vi "Write Used DAQChannels.vi"(8 "error in (no error)":errorcluster, 10 "Used DAQChannels":tag[](array[tag]), 11 "SequencerConfig in":refnum<class "SequencerConfig.lvclass">) -> (0 "error out":errorcluster, 3 "SequencerConfig out":refnum<class "SequencerConfig.lvclass">)   [LabVIEW 2015, in "Sequencer.lvlib" / "SequencerConfig.lvclass"]
uses:
  SequencerConfig.lvclass
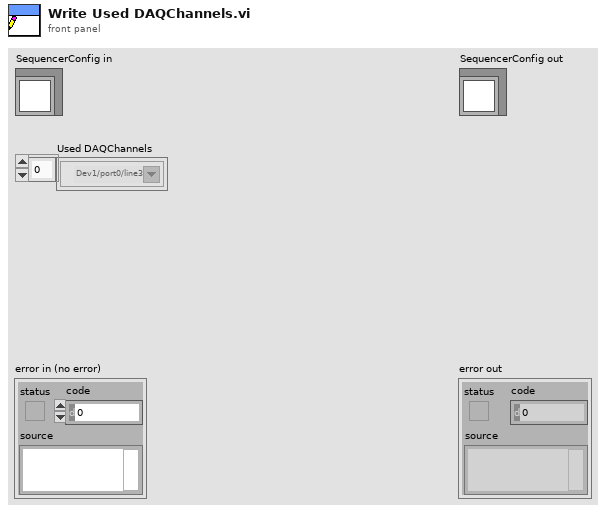
[diagram p1: front panel]
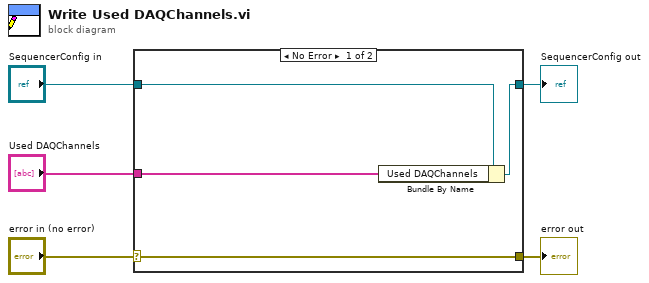
[diagram p0: block diagram]
diagram:
  n1 = case shown="No Error" "error in (no error)" {
    selector: "error in (no error)" -> [w9 w10]
    tunnel: [w9 w10] -> w4
    tunnel: [w7 w11] -> w2
    tunnel: "SequencerConfig in" -> [w8 w11]
    tunnel: "Used DAQChannels" -> [w6 _]
    frame No Error {
      n2 = Bundle By Name(cluster=w8, "Used DAQChannels"=w6) -> (w7:refnum<class "SequencerConfig.lvclass">)
    }
    frame Error {
    }
  }
  "error out" <- w4
  "SequencerConfig out" <- w2
